vi "DDS Set RAM Profile.vi"(0 "DDS ref in":T2={"NI USB-8451 device reference"="", "DIO port"=0, "Serial Clock Rate [kHz]"=1000}, 1 "Start Address":u16, 4 "End Address":u16, 5 "error in (no error)":errorcluster, 6 "RAM mode":T1, 7 "channel number (1)":u8=1 min=1 max=4 step=1, 9 "Zero-crossing":bool, 11 "No Dwell High":bool, 12 "Profile (0)":u8, 13 "Step Rate":u16) -> (14 "DDS ref out":T2={"NI USB-8451 device reference"="", "DIO port"=0, "Serial Clock Rate [kHz]"=1000}, 15 "Write Data":u8[](array[numeric]), 19 "error out":errorcluster)   [LabVIEW 2013, in "DDS.lvlib"]
doc: "Program the RAM Profiles so they are ready to use the RAM settings."
uses:
  DDS.lvlib
  Controls/DDS Box Device Reference.ctl
  <vilib>/ni845x/ni845x.llb/ni845xControl.ctl
  Controls/DDS RAM Mode.ctl
  Controls/AD9910 registers.ctl
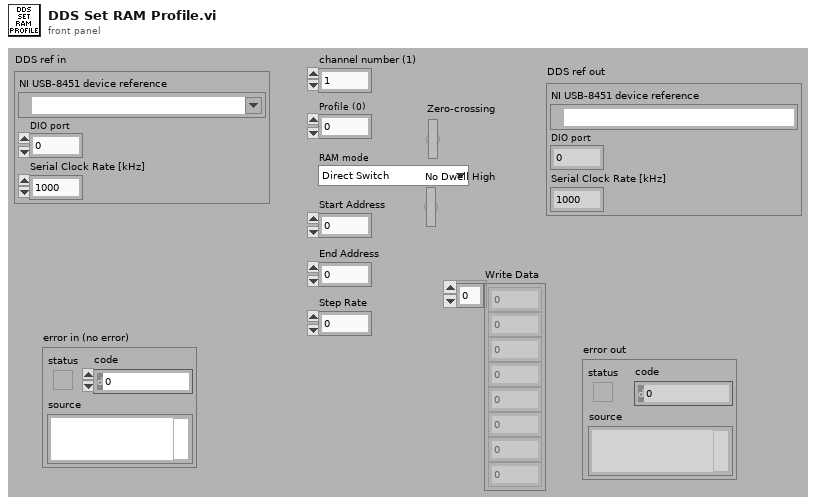
[diagram p1: front panel]
types:
  T1 = typedef "DDS.lvlib/DDS RAM mode.ctl" = enum16{"Direct Switch", "Ramp Up", "Bidirectional Ramp", "Continuous Bidirectional Ramp", "Continuous Recirculate", "Direct Switch 2", "Direct Switch 3", "Direct Switch 4"}
  T2 = typedef "DDS.lvlib/DDS Box Device Reference.ctl" = cluster{"NI USB-8451 device reference":T3, "DIO port":u8, "Serial Clock Rate [kHz]":u16}
  T3 = typedef "ni845xControl.ctl" = refnum<k21>
  T4 = typedef "DDS.lvlib/AD9910 registers.ctl" = enum16{"CFR1", "CFR2", "CFR3", "Auxiliary DAC Control", "I/0 Update Rate", "Frequency Tuning Word", "Phase Offset Word", "Amplitude Scale Factor", "Multichip Sync", "Digital Ramp Limit", "Digital Ramp Step Size", "Digital Ramp Rate", "Single Tone Profile 0", "Single Tone Profile 1", "Single Tone Profile 2", "Single Tone Profile 3", "Single Tone Profile 4", "Single Tone Profile 5", "Single Tone Profile 6", "Single Tone Profile 7", "RAM Profile 0", "RAM Profile 1", "RAM Profile 2", "RAM Profile 3", "RAM Profile 4", "RAM Profile 5", "RAM Profile 6", "RAM Profile 7", "RAM"}
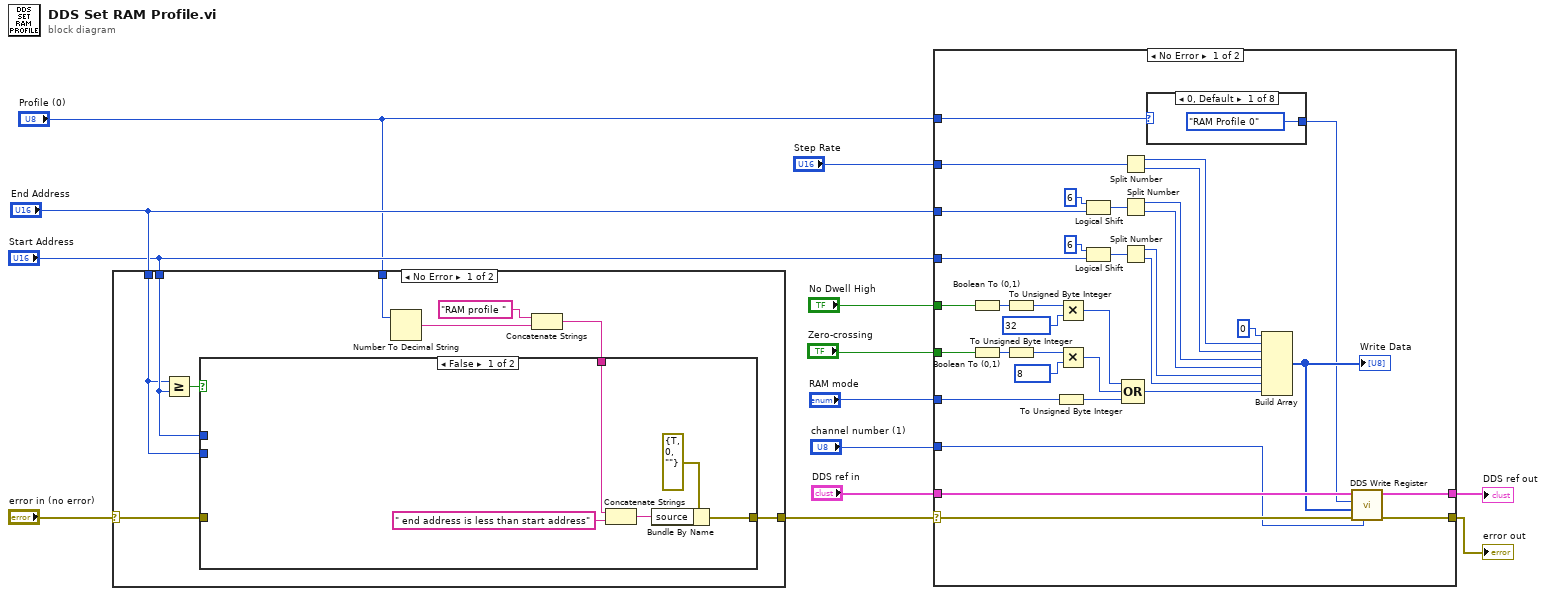
[diagram p0: block diagram]
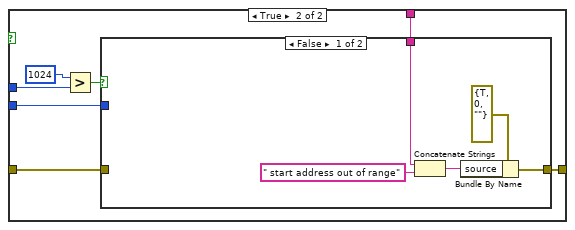
[diagram p2: hidden frame]
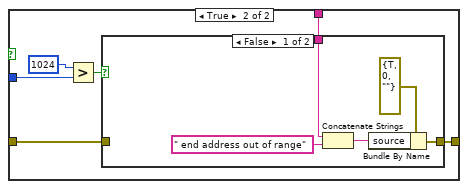
[diagram p3: hidden frame]
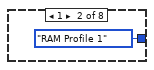
[diagram p6: hidden frame]
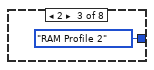
[diagram p7: hidden frame]
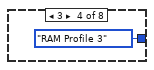
[diagram p8: hidden frame]
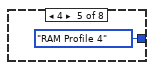
[diagram p9: hidden frame]
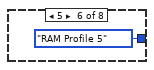
[diagram p10: hidden frame]
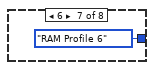
[diagram p11: hidden frame]
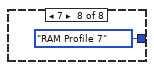
[diagram p12: hidden frame]
diagram:
  n1 = case shown="No Error" "error in (no error)" {
    selector: "error in (no error)" -> [w14 w52]
    tunnel: [w22 w52] -> w13
    tunnel: "Profile (0)" -> [w20 _]
    tunnel: "Start Address" -> [w19 _]
    tunnel: "End Address" -> [w18 _]
    frame No Error {
      n2 = Greater Or Equal?(x=w18, y=w19) -> (x >= y?=w21:bool)
      n3 = Number To Decimal String(number=w20) -> (decimal integer string=w16:string)  [unwired: 1 in]
      n4 = Concatenate Strings("RAM profile " ("source"), w16) -> (w15:string)
      n5 = case shown="False" w21 {
        tunnel: [w26 w30] -> w22
        tunnel: w14 -> [_ w28]
        tunnel: w15 -> [w23 w29]
        tunnel: w19 -> [_ w33]
        tunnel: w18 -> [_ w31]
        frame False {
          n6 = Concatenate Strings(w23, " end address is less than start address" ("source")) -> (w25:string)
          n7 = Bundle By Name(cluster=errorcluster {"status"=TRUE, "code"=0, "source"=""} ("error in (no error)"), "source"=w25) -> (w26:errorcluster)
        }
        frame True {
          n8 = Greater?(x=u16 1024 ("upper limit"), y=w33) -> (0:w32:bool)
          n9 = case shown="False" w32 {
            tunnel: w31 -> [_ w44]
            tunnel: [w36 w42] -> w30
            tunnel: w29 -> [w35 w41]
            tunnel: w28 -> [_ w40]
            frame False {
              n10 = Concatenate Strings(w35, " start address out of range" ("string")) -> (w39:string)
              n11 = Bundle By Name(cluster=errorcluster {"status"=TRUE, "code"=0, "source"=""} ("error in (no error)"), "source"=w39) -> (w36:errorcluster)
            }
            frame True {
              n12 = Greater?(x=u16 1024 ("upper limit"), y=w44) -> (0:w43:bool)
              n13 = case shown="False" w43 {
                tunnel: [w48 w51] -> w42
                tunnel: w41 -> [w47 _]
                tunnel: w40 -> [_ w51]
                frame False {
                  n14 = Concatenate Strings(w47, " end address out of range" ("string")) -> (w49:string)
                  n15 = Bundle By Name(cluster=errorcluster {"status"=TRUE, "code"=0, "source"=""} ("error in (no error)"), "source"=w49) -> (w48:errorcluster)
                }
                frame True {
                }
              }
            }
          }
        }
      }
    }
    frame Error {
    }
  }
  n16 = case shown="No Error" w13 {
    selector: w13 -> [w56 w96]
    tunnel: [w57 w96] -> w11
    tunnel: "Profile (0)" -> [w60 _]
    tunnel: "DDS ref in" -> [w58 w97]
    tunnel: [w59 w97] -> w12
    tunnel: "channel number (1)" -> [w55 _]
    tunnel: "RAM mode" -> [w74 _]
    tunnel: "Zero-crossing" -> [w82 _]
    tunnel: "No Dwell High" -> [w84 _]
    tunnel: "Start Address" -> [w75 _]
    tunnel: "End Address" -> [w64 _]
    tunnel: "Step Rate" -> [w78 _]
    frame No Error {
      n17 = Boolean To (0,1)(Boolean=w84) -> (0, 1=w85:i16)
      n18 = Boolean To (0,1)(Boolean=w82) -> (0, 1=w86:i16)
      n19 = To Unsigned Byte Integer(number=w85) -> (unsigned 8bit integer=w72:u8)
      n20 = To Unsigned Byte Integer(number=w86) -> (unsigned 8bit integer=w73:u8)
      n21 = To Unsigned Byte Integer(number=w74) -> (unsigned 8bit integer=w70:u8)
      n22 = Multiply(x=w72, y=u8 32) -> (x*y=w71:u8)
      n23 = Multiply(x=w73, y=u8 8) -> (x*y=w61:u8)
      n24 = Logical Shift(y=i8 6, x=w64) -> (x << y=w66:u16)
      n25 = Logical Shift(y=i8 6, x=w75) -> (x << y=w67:u16)
      n26 = Split Number(x=w78) -> (hi(x)=w76:u8, lo(x)=w77:u8)
      n27 = Split Number(x=w66) -> (hi(x)=w62:u8, lo(x)=w63:u8)
      n28 = Split Number(x=w67) -> (hi(x)=w80:u8, lo(x)=w81:u8)
      n29 = Compound Arithmetic op=OR(w71, w61, w70) -> (w69:u8)
      n30 = case shown="0, Default" w60 {
        tunnel: [AD9910_registers."RAM Profile 0" ("Register") AD9910_registers."RAM Profile 1" ("Register") AD9910_registers."RAM Profile 2" ("Register") AD9910_registers."RAM Profile 3" ("Register") AD9910_registers."RAM Profile 4" ("Register") AD9910_registers."RAM Profile 5" ("Register") AD9910_registers."RAM Profile 6" ("Register") AD9910_registers."RAM Profile 7" ("Register")] -> w53
        frame 0, Default {
        }
        frame 1 {
        }
        frame 2 {
        }
        frame 3 {
        }
        frame 4 {
        }
        frame 5 {
        }
        frame 6 {
        }
        frame 7 {
        }
      }
      n31 = Build Array(u8 0 ("element"), w76, w77, w62, w63, w80, w81, w69) -> (w54:u8[])
      "Write Data" <- w54
      n32 = call "DDS Write Register.vi"("channel number (1)"=w55, "error in (no error)"=w56, "Write Data"=w54, "Register"=w53, "DDS ref in"=w58) -> ("error out"=w57:errorcluster, "DDS ref out"=w59:T2)  [unwired: 4 in, 1 out]
    }
    frame Error {
    }
  }
  "error out" <- w11
  "DDS ref out" <- w12
